vi "Convert num array to string.vi"(3 "Num. values":dbl[](array[numeric]) format="%.6f", 4 "No. of digits":i16=4) -> (14 "Output string":string)   [LabVIEW 2026]
doc: "This VI converts an array of numerical values to a space separated output string. The difference to LabVIEW's native Array to Spreadsheet String function is that no carriage return or newline is added."
panel:
  # "This vi converts an array of numerical values to a space separated\noutput string. The difference to LabVIEW's native Array to Spread-\nsheet String function is that no carriage return or newline is added."
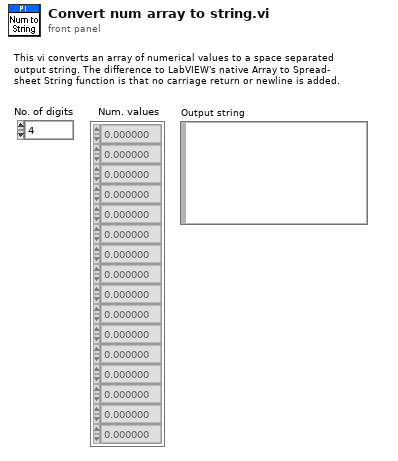
[diagram p1: front panel]
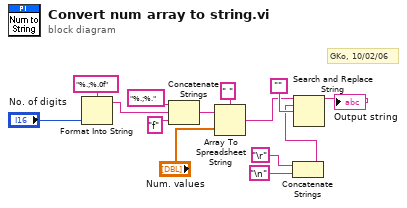
[diagram p0: block diagram]
diagram:
  # "GKo, 10/02/06"
  n1 = Format Into String(format string="%.;%.0f" ("Format String"), "No. of digits") -> (resulting string=w3:string)  [unwired: 2 in, 1 out]
  n2 = Concatenate Strings("%.;%." ("Format String"), w3, "f" ("Format String")) -> (w1:string)
  n3 = Array To Spreadsheet String(delimiter (Tab)=" ", array="Num. values", 3:w1) -> (spreadsheet string=w11:string)
  n4 = Concatenate Strings("\r", "\n") -> (w8:string)
  n5 = Search and Replace String(input string=w11, search string=w8, replace string="" ("replace string (\"\")")) -> (result string=→"Output string":string)  [unwired: 1 in, 7 out]
